vi "Get Result.vi"(4 "Controller name":string, 6 "Last request":bool, 8 "error in (no error)":errorcluster, 11 "VI Server Recorder in":refnum<class "VI Server Recorder.lvclass">) -> (0 "error out":errorcluster, 2 "Result":refnum<class "Acquired Result.lvclass">, 3 "VI Server Recorder out":refnum<class "VI Server Recorder.lvclass">)   [LabVIEW 2021, in "VI Server Recorder.lvclass"]
uses:
  VI Server Recorder.lvclass
  C:/GitHub/LabActor/Worker/Worker Actor.lvclass
  NHMFL_Core/Libraries/Instruments/Results/Acquired Result/Acquired Result.lvclass
  Worker/Worker Actor/Worker Actor.lvclass/Worker Actor.ctl
  <vilib>/express/express signal manip/GetorSetDDTAttributes/Shared VIs/TimeType.ctl
  NHMFL_Core/Libraries/Instruments/Results/Acquired Result/Acquired Result.lvclass/Acquired Result.ctl
  Worker/Worker Actor/Read Cycle period.vi
  NHMFL_Core/Libraries/Instruments/Results/Acquired Result/Write Channels.vi
  NHMFL_Core/Libraries/Instruments/Results/Acquired Result/Write Sender.vi
  NHMFL_Core/Libraries/Instruments/Results/Acquired Result/Write Group.vi
  NHMFL_Core/Libraries/Instruments/Results/Acquired Result/Write Final.vi
  <vilib>/express/express signal manip/GetorSetDDTAttributes/Shared VIs/TimeMode Enum to Boolean.vi
  <vilib>/express/express shared/transition.llb/Dynamic To Waveform Array.vi
  <vilib>/express/express signal manip/GetorSetDDTAttributes/Set DDT Attributes/SetT0.vi
  <vilib>/express/express shared/transition.llb/Waveform Array To Dynamic.vi
  Worker/Worker Actor/Worker Actor.lvclass
  <vilib>/express/express signal manip/GetorSetDDTAttributes/Set DDT Attributes/Set DDT Properties.xnode
  <vilib>/express/express signal manip/GetorSetDDTAttributes/Shared VIs/GetSetShared.lvlib
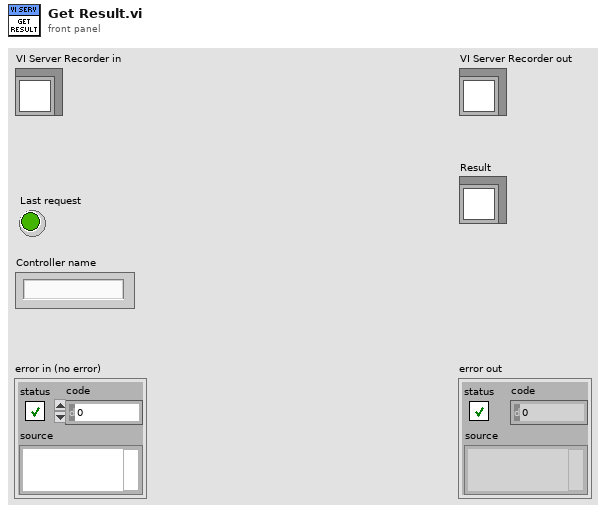
[diagram p1: front panel]
types:
  T1 = typedef "VI Server Configuration.ctl" = cluster{"Machine name (\"\":  open local reference)":string, "Port number (3363)":u16, "Control names":string[], "VI  name":string}
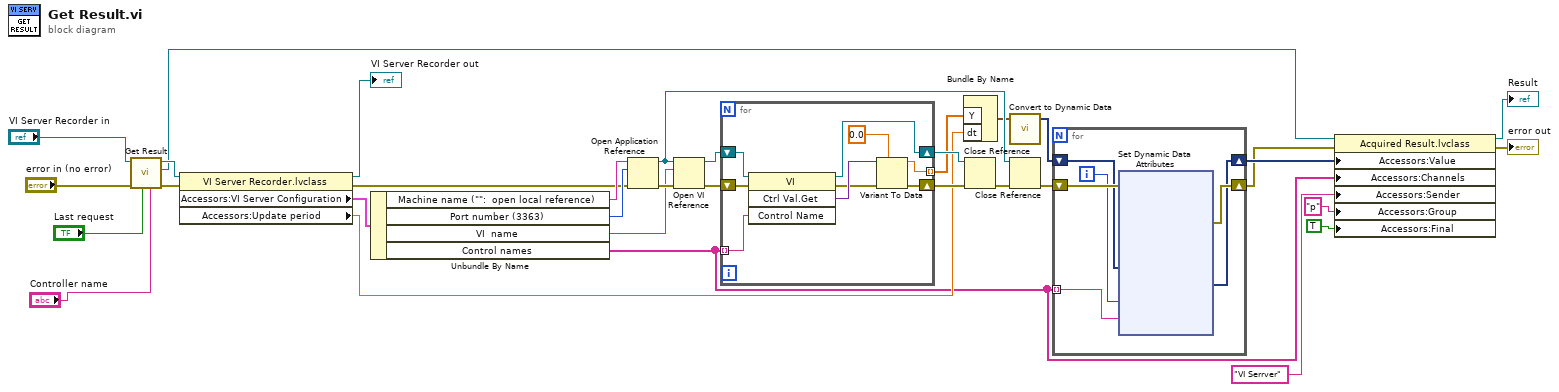
[diagram p0: block diagram]
diagram:
  n1 = call-parent "Get Result.vi"("Controller name"="Controller name", "Last request"="Last request", "error in (no error)"="error in (no error)", "Worker in"="VI Server Recorder in") -> ("error out"=w33:errorcluster, "Result"=w12:refnum<class "Acquired Result.lvclass">, "Worker out"=w27:refnum<class "VI Server Recorder.lvclass">)  [unwired: 5 in]
  n2 = property class="VI Server Recorder.lvclass"(reference=w27, error in=w33) -> (reference out=→"VI Server Recorder out":refnum<class "VI Server Recorder.lvclass">, error out=w21:errorcluster, "Accessors:VI Server Configuration"=w25:T1, "Accessors:Update period"=w14:dbl)
  n3 = Unbundle By Name(w25) -> ("Machine name (\"\":  open local reference)"=w24:string, "Port number (3363)"=w23:u16, "VI  name"=w22:string, "Control names"=w7:string[])
  n4 = Open Application Reference(8:w21, 10:w23, 11:w24) -> (0:w29:errorcluster, 3:w17:refnum<vi>)  [unwired: 1 in]
  n5 = Open VI Reference(application reference (local)=w17, vi path=w22, error in (no error)=w29) -> (vi reference=w28:refnum<vi>, error out=w20:errorcluster)  [unwired: 3 in]
  n6 = for {
    tunnel: w7 -> [w40] mode=indexing
    shift-right: [w36] -> w19
    shift-left: w20 -> [w41]
    shift-right: [w39] -> w18
    shift-left: w28 -> [w42]
    tunnel: [w35] -> w15 mode=indexing
    n7 = invoke class="VI" method="Ctrl Val.Get"(reference=w42, error in=w41, "Control Name"=w40) -> (reference out=w39:refnum<vi>, error out=w37:errorcluster, "Get Control Value Variant"=w38:variant)  [unwired: 1 in, 1 out]
    n8 = Variant To Data(error in=w37, type=0.0, Variant=w38) -> (data=w35:dbl, error out=w36:errorcluster)
  }
  n9 = Bundle By Name("Y"=w15, "dt"=w14) -> (w13:waveform(dbl))  [unwired: 1 in]
  n10 = Close Reference(reference=w18, error in (no error)=w19) -> (error out=w16:errorcluster)
  n11 = call "Convert to Dynamic Data"("Waveform"=w13) -> ("Dynamic Data Type"=w9:dynamicdata)  [unwired: 3 in]
  n12 = Close Reference(reference=w17, error in (no error)=w16) -> (error out=w10:errorcluster)
  n13 = for {
    tunnel: w7 -> [w43] mode=indexing
    shift-right: [w47] -> w2
    shift-left: w10 -> [w48]
    shift-right: [w45] -> w8
    shift-left: w9 -> [w46]
    i -> [w44]
    n14 = xnode "Set Dynamic Data Attributes"("Signals In"=w46, "Signal Index"=w44, "Signal Name"=w43, "error in"=w48) -> ("Signals Out"=w45:dynamicdata, "error out"=w47:errorcluster)  [unwired: 2 in]
  }
  n15 = property class="Acquired Result.lvclass"(reference=w12, error in=w2, "Accessors:Value"=w8, "Accessors:Channels"=w7, "Accessors:Sender"="VI Serrver" ("String"), "Accessors:Group"="p" ("Group"), "Accessors:Final"=TRUE ("Final")) -> (reference out=→"Result":refnum<class "Acquired Result.lvclass">, error out=→"error out":errorcluster)
